vi "PSP-603_Serial.vi"(5 "Command":string="L\r", 6 "Emergency":bool, 8 "error in (no error)":errorcluster, 9 "Read Buffer?":bool, 11 "VISA resource name":refnum<visa-resource-name>="COM1") -> (0 "error out":errorcluster, 3 "Response":string, 10 "bytes read":u32)   [LabVIEW 2021]
doc: "This example performs a serial port write and a serial port read. The parameters set for the serial port must match the parameters of the connected instrument or device. The VISA Configure Serial Port VI sets the configuration parameters. The front panel displays the controls used to configure the basic parameters, such as baud rate, data bits, and parity. The VI passes the VISA resource name to other VIs that perform operations on that VISA resource. The VISA Write function sends a command to the serial device and the VISA Read function returns data based on the command. The VISA Close function then closes the reference to the serial device. It is important to close the reference; otherwise, further communication through that port might not be possible."
uses:
  <vilib>/Instr/_visa.llb/VISA Configure Serial Port (Instr).vi
panel:
  in  "Serial Settings":T1={"baud rate"=2400, "data bits"=8, "parity"=enum."None", "stop bits"=10, "flow control"=0} {"flow control" items=["None"=0, "XON/XOFF"=1, "RTS/CTS"=2, "DTR/DSR"=4]; "stop bits" items=["1.0"=10, "1.5"=15, "2.0"=20]; "data bits" min=5 max=8 step=1; "baud rate" items=["75"=75, "110"=110, "134"=134, "150"=150, "300"=300, "600"=600, "1200"=1200, "1800"=1800, "2400"=2400, "4800"=4800, "7200"=7200, "9600"=9600, "14400"=14400, "19200"=19200, "28800"=28800, "38400"=38400, "56000"=56000, "57600"=57600, "115200"=115200, "128000"=128000, "230400"=230400]}
  out "specific error cleared?":bool
  in  "delay before read (ms)":u32=500
  # "L<CR> The L query returns all the status values of the power supply.\n\nVvv.vvAa.aaaWwww.wUuuIi.iiPpppFf1f2f3f4f5f6<CR>\n\nV:Voltage Unit            uu:Voltage limit value    f1 : Relay Status:         ( 0:Off 1:On )                       \nvv.vv:Voltage Value    I:Current limit unit        f2 :Temperature Status  ( 0:Normal 1:Overtemp )   \nA:Current Unit                  i.ii:Current limit value    f3:Step mode:                  ( 0:Coarse 1:Fine ) \na.aaa:Current value           P:Power limit unit               f4:Scroll wheel status:      ( 0:Locked 1:Unlocked ) \nW:Power unit                               ppp:Power limit value     f5:Remote Status:             ( 0:Normal 1:Remote ) \nwww.w:Power value        F:Status Byte Character      f6:6 : Lock Status:             ( 0:Unloced 1:Locked ) \nU:Voltage limit unit"
  # "Serial port communication codes;\n\n1 KOE<CR> The KOE command turns the output On.   \n\n2- KOD<CR> The KOD command turns the output Off.  \n\n3-SV 10.50<CR>  Sets the voltage output to 10.5V.\n\n4-SU 11<CR>     Sets the voltage limit to 11 V.\n\n5-A<CR> Returns the current output.\n\n6-V<CR> Returns the voltage output..\n\n7-W<CR> Returns the load output.\n\n8-SI 1 .10<CR>    Sets the current limit to 1.10A.\n\n9-SP 100<CR>  Sets the power limit to 100W.\n\n10-EEP<CR>   Save settings to memory."
  # "PSP-603"
  # "2400 boud rate"
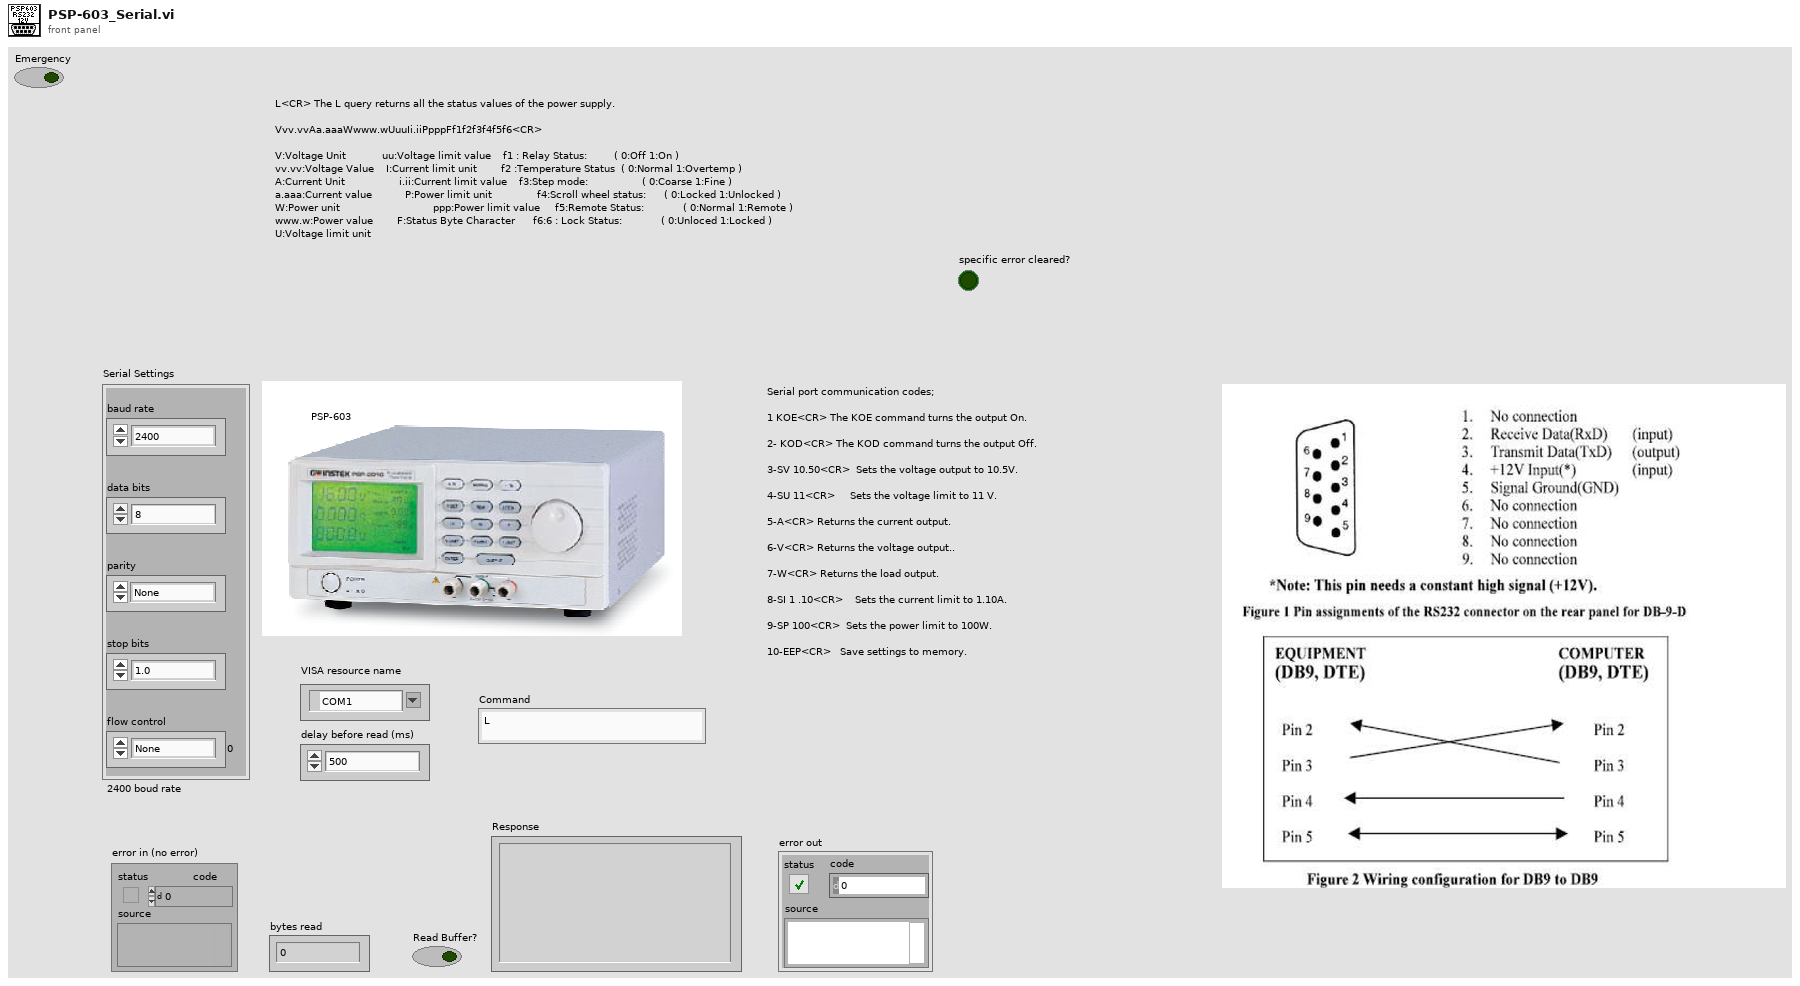
[diagram p1: front panel]
types:
  T1 = cluster{"baud rate":u32, "data bits":u16, "parity":enum16{"None", "Odd", "Even", "Mark", "Space"}, "stop bits":u16, "flow control":u16}
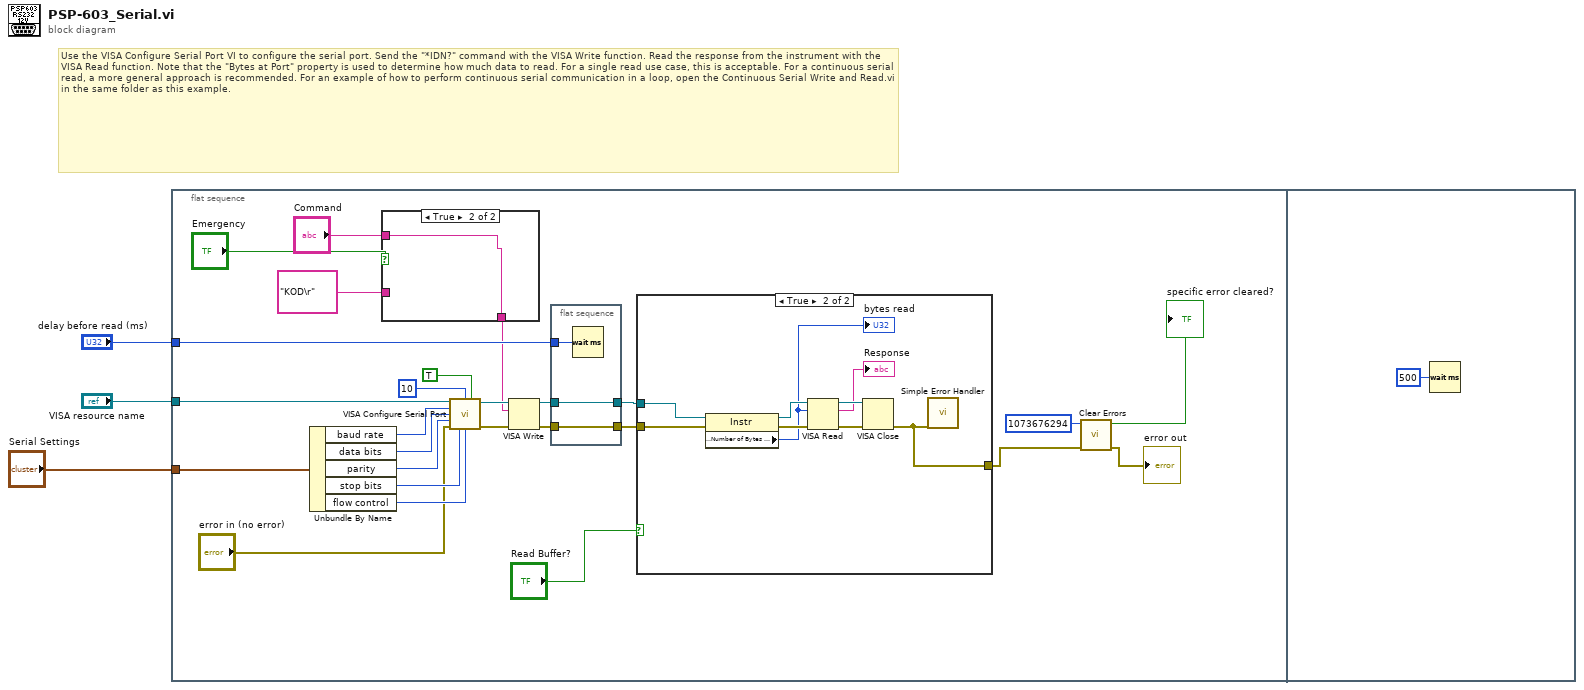
[diagram p0: block diagram]
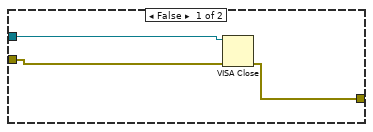
[diagram p3: hidden frame]
diagram:
  # "Use the VISA Configure Serial Port VI to configure the serial port. Send the \"*IDN?\" command with the VISA Write function. Read the response from the instrument with the VISA Read function. Note that the \"Bytes at Port\" property is used to determine how much data to read. For a single read use case, this is acceptable. For a continuous serial read, a more general approach is recommended. For an example of how to perform continuous serial communication in a loop, open the Continuous Serial Write and Read.vi in the same folder as this example."
  n1 = flat-sequence {
    tunnel: "VISA resource name" -> [w29]
    tunnel: "delay before read (ms)" -> [w22]
    tunnel: "Serial Settings" -> [w21]
    frame #0 {
      n2 = Unbundle By Name(w21) -> ("baud rate"=w20:u32, "data bits"=w19:u16, "parity"=w18:enum16{"None", "Odd", "Even", "Mark", "Space"}, "stop bits"=w17:u16, "flow control"=w16:u16)
      n3 = case shown="True" "Emergency" {
        tunnel: [w30 w31] -> w7
        tunnel: "Command" -> [_ w31]
        tunnel: "KOD\r" ("Command") -> [w30 _]
        frame False {
        }
        frame True {
        }
      }
      n4 = call-poly "VISA Configure Serial Port"("VISA resource name"=w29, "termination char\n(0xA = '\\n' = LF)"=u8 10 ("termination char\n(0xA = '\\n' = LF)"), "Enable Termination\nChar (T)"=TRUE ("Enable Termination\nChar (T)"), "baud rate (9600)"=w20, "data bits (8)"=w19, "parity (0:none)"=w18, "error in (no error)"="error in (no error)", "stop bits (10: 1 bit)"=w17, "flow control (0:none)"=w16) -> ("VISA resource name out"=w27:refnum<visa-resource-name>, "error out"=w28:errorcluster)  [unwired: 1 in, 4 out]
      n5 = VISA Write(VISA resource name=w27, write buffer=w7, error in (no error)=w28) -> (VISA resource name out=w24:refnum<visa-resource-name>, error out=w26:errorcluster)  [unwired: 1 out]
      n6 = flat-sequence {
        tunnel: w26 -> [w45]
        tunnel: [w45] -> w25
        tunnel: w24 -> [w44]
        tunnel: [w44] -> w23
        tunnel: w22 -> [w46]
        frame #0 {
          n7 = Wait (ms)(milliseconds to wait=w46) -> ()  [unwired: 1 out]
        }
      }
      n8 = case shown="True" "Read Buffer?" {
        tunnel: w25 -> [w33 w41]
        tunnel: w23 -> [w34 w40]
        tunnel: [w32 w35] -> w10
        frame False {
          n9 = VISA Close(VISA resource name=w34, error in (no error)=w33) -> (error out=w32:errorcluster)
        }
        frame True {
          n10 = property class="Instr"(reference=w40, error in=w41) -> (reference out=w39:refnum<visa-resource-name>, error out=w38:errorcluster, "Serial Settings:Number of Bytes at Serial Port"=w36:u32)
          "bytes read" <- w36
          n11 = VISA Read(VISA resource name=w39, byte count=w36, error in (no error)=w38) -> (VISA resource name out=w42:refnum<visa-resource-name>, read buffer=→"Response":string, error out=w43:errorcluster)  [unwired: 1 out]
          n12 = VISA Close(VISA resource name=w42, error in (no error)=w43) -> (error out=w35:errorcluster)
          n13 = call <vilib>:"Simple Error Handler.vi"("error in (no error)"=w35) -> ()  [unwired: 1 in, 8 out]
        }
      }
      n14 = call <vilib>:"Clear Errors.vi"("error in (no error)"=w10, "specific error code to clear (0: all)"=1073676294) -> ("error out"=→"error out":errorcluster, "specific error cleared?"=→"specific error cleared?":bool)  [unwired: 4 in]
    }
    frame #1 {
      n15 = Wait (ms)(milliseconds to wait=u32 500) -> ()  [unwired: 1 out]
    }
  }
